vi "Excercise 4-1.vi"(8 "error in (no error)":errorcluster, 9 "Min Temp":dbl, 10 "Max Temp":dbl, 11 "Current Temp":dbl) -> (0 "error out":errorcluster, 1 "Warning?":bool, 2 "Warning Text":string)   [LabVIEW 2014]
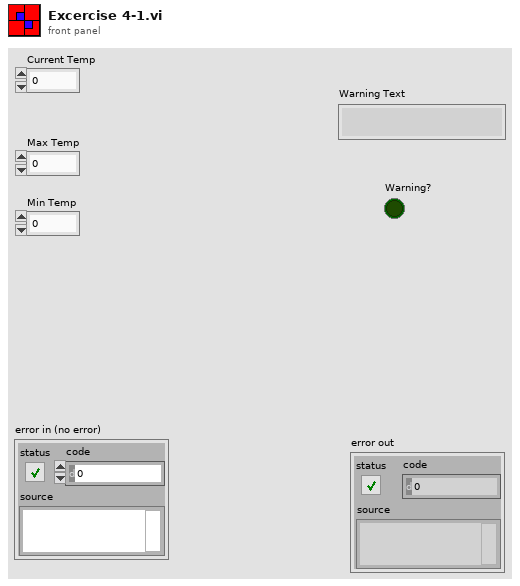
[diagram p1: front panel]
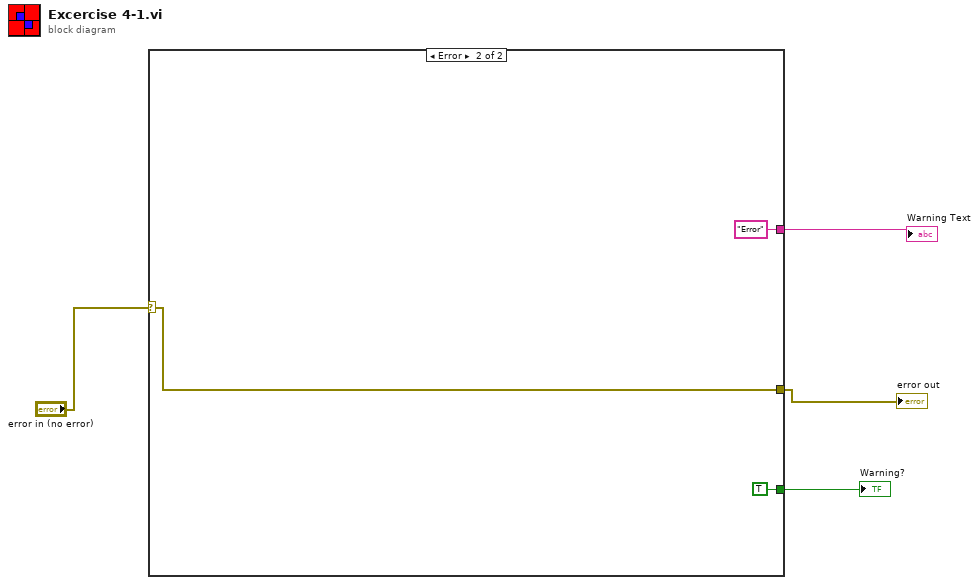
[diagram p0: block diagram]
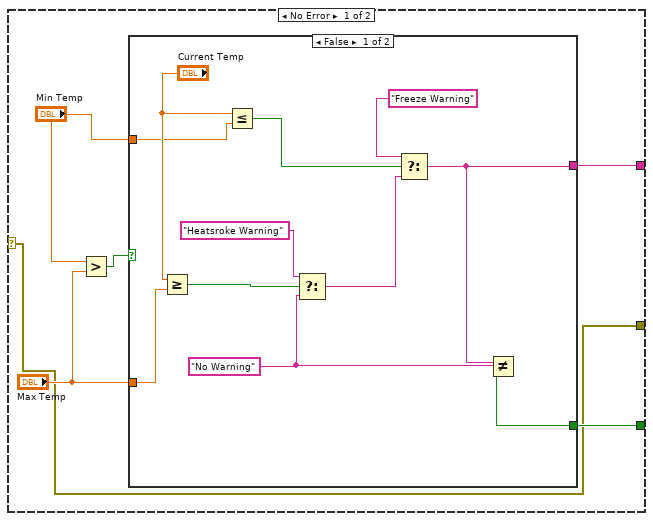
[diagram p2: hidden frame]
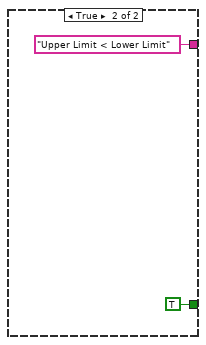
[diagram p3: hidden frame]
diagram:
  n1 = case shown="Error" "error in (no error)" {
    selector: "error in (no error)" -> [w5 w26]
    tunnel: [w10 TRUE] -> w4
    tunnel: [w9 "Error"] -> w3
    tunnel: [w5 w26] -> w1
    frame No Error {
      n2 = Greater?(x="Min Temp", y="Max Temp") -> (0:w6:bool)
      n3 = case shown="False" w6 {
        tunnel: [w14 TRUE] -> w10
        tunnel: [w13 "Upper Limit < Lower Limit"] -> w9
        tunnel: "Min Temp" -> [w12 _]
        tunnel: "Max Temp" -> [w11 _]
        frame False {
          w15 = "No Warning"
          n4 = Greater Or Equal?(x="Current Temp", y=w11) -> (x >= y?=w20:bool)
          n5 = Less Or Equal?(x="Current Temp", y=w12) -> (x <= y?=w18:bool)
          n6 = Select(t="Heatsroke Warning", s=w20, f=w15) -> (s? t:f=w16:string)
          n7 = Select(t="Freeze Warning", s=w18, f=w16) -> (s? t:f=w13:string)
          n8 = Not Equal?(x=w13, y=w15) -> (x != y?=w14:bool)
        }
        frame True {
        }
      }
    }
    frame Error {
    }
  }
  "Warning Text" <- w3
  "Warning?" <- w4
  "error out" <- w1
